vi "Read Instrument.vi"(0 "Instrument Prop":T1 {"Private"."Offset" format="%^_3e"; "Private"."Scale Factors" format="%^_3e"}, 1 "Array":dbl[](array[numeric])) -> (2 "Instrument Prop 2":T1 {"Private"."Offset" format="%^_3e"; "Private"."Scale Factors" format="%^_3e"}, 3 "Array 2":dbl[](array[numeric]), 4 "Stop":bool)   [LabVIEW 2021]
uses:
  New NML Data Acq/Sub Controls/Instrument Properties.ctl
  New NML Data Acq/Sub Controls/Public.ctl
  New NML Data Acq/Sub Controls/Private.ctl
  New NML Data Acq/Sub Controls/Instrument Ref.ctl
  New NML Data Acq/Sub Controls/SystemCheckBox-resize.ctl
  New NML Data Acq/Sub Controls/Instrument Actions.ctl
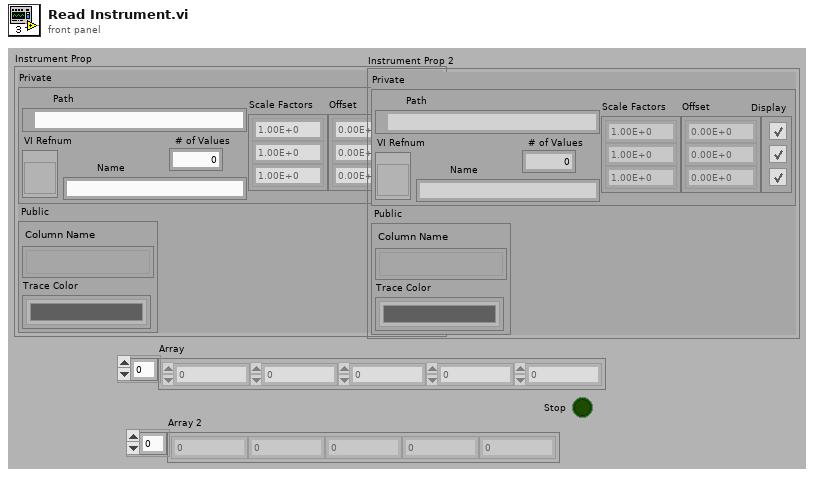
[diagram p1: front panel]
types:
  T1 = typedef "Instrument Properties.ctl" = cluster{"Public":T2, "Private":T3}
  T2 = typedef "Public.ctl" = cluster{"Column Name":string[], "Trace Color":u32[]}
  T3 = typedef "Private.ctl" = cluster{"Path":path, "VI Refnum":T4, "Name":string, "# of Values":i32, "Scale Factors":dbl[], "Display":T5[], "Offset":dbl[]}
  T4 = typedef "Instrument Ref.ctl" = refnum<vi>
  T5 = typedef "SystemCheckBox-resize.ctl" = bool
  T6 = typedef "Instrument Actions.ctl" = enum16{"Scan", "Identify", "New", "Configure", "Initialize", "Test", "Read", "Close"}
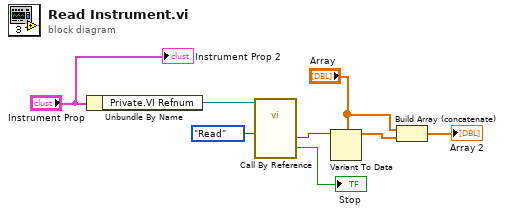
[diagram p0: block diagram]
diagram:
  n1 = Unbundle By Name("Instrument Prop") -> ("Private.VI Refnum"=w7:T4)
  n2 = call-by-ref "?"(reference=w7, "Action"=Instrument_Actions."Read") -> ("Output"=w5:variant, "Stop"=→"Stop":bool)  [unwired: 6 in, 2 out]
  n3 = Variant To Data(type="Array", Variant=w5) -> (data=w2:dbl[])  [unwired: 1 in, 1 out]
  n4 = Build Array (concatenate)("Array", w2) -> (→"Array 2":dbl[])
  "Instrument Prop 2" <- "Instrument Prop"
